vi "Get Highest Sub-Index.vi"(8 "Error In":errorcluster, 11 "reference in":refnum<class "OD Entry.lvclass">) -> (0 "Error Out":errorcluster, 2 "Highes Sub-Index":u8, 3 "reference out":refnum<class "OD Entry.lvclass">)   [LabVIEW 2024, in "EDS.lvlib" / "OD Entry.lvclass"]
doc: "Return max indicated subindex, or null if not array or record"
uses:
  OD Entry.lvclass
  OD Entry.lvclass/OD Entry.ctl
  Object Type.ctl
  EDS.lvlib
  Object Type/Object Type Base.lvclass
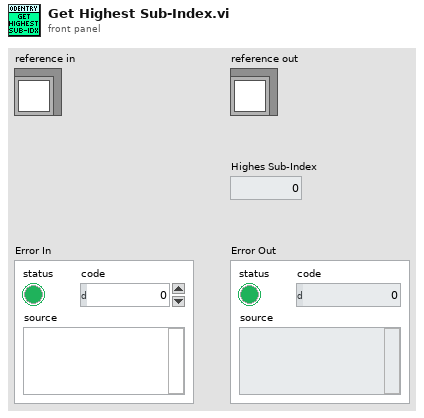
[diagram p1: front panel]
types:
  T1 = typedef "EDS.lvlib/Object Type.ctl" = u8
  T2 = typedef "EDS.lvlib/OD Entry.lvclass/ObjectAttributes.ctl" = cluster{"Index":u16, "ObjectType":refnum<class "Object Type Base.lvclass">, "Denotation":string, "Count":u8, "ObjExtend":u8, "PDOtype":T3, "Label":string, "Description":string, "Sub-Entries":map{u8, refnum<class "OD Sub-Entry.lvclass">}}
  T3 = typedef "EDS.lvlib/PDO Mapping Type.ctl" = enum16{"NO", "OPTIONAL", "RPDO", "TPDO", "DEFAULT"}
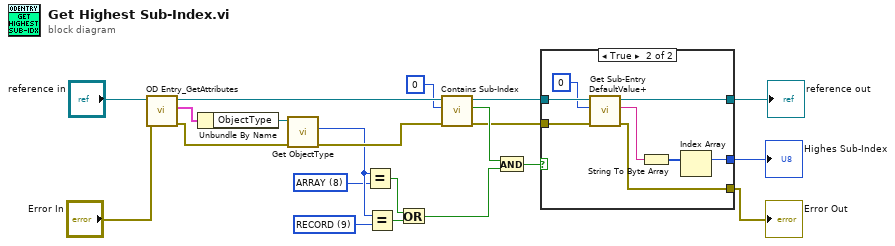
[diagram p0: block diagram]
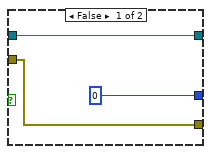
[diagram p2: hidden frame]
diagram:
  w1 = T1 9 items=["NULL"=0, "DOMAIN"=2, "DEFTYPE"=5, "DEFSTRUCT"=6, "VAR"=7, "ARRAY"=8, "RECORD"=9] ("ObjectType")
  w2 = T1 8 items=["NULL"=0, "DOMAIN"=2, "DEFTYPE"=5, "DEFSTRUCT"=6, "VAR"=7, "ARRAY"=8, "RECORD"=9] ("ObjectType")
  n1 = call "OD Entry_GetAttributes.vi"("Error In"="Error In", "reference in"="reference in") -> ("Error Out"=w5:errorcluster, "Data"=w18:T2, "reference out"=w19:refnum<class "OD Entry.lvclass">)  [unwired: 6 in, 1 out]
  n2 = Unbundle By Name(w18) -> ("ObjectType"=w16:refnum<class "Object Type Base.lvclass">)
  n3 = call-dynamic "Get ObjectType.vi"("error in"=w5, "Object Type in"=w16) -> ("error out"=w4:errorcluster, "ObjectType"=w3:T1)  [unwired: 6 in, 2 out]
  n4 = Equal?(x=w3, y=w2) -> (x = y?=w17:bool)
  n5 = Equal?(x=w3, y=w1) -> (x = y?=w13:bool)
  n6 = Or(x=w17, y=w13) -> (x .or. y?=w11:bool)
  n7 = call "Contains Sub-Index.vi"("Error In"=w4, "Sub-Index"=u16 0, "reference in"=w19) -> ("Error Out"=w7:errorcluster, "Contains?"=w12:bool, "reference out"=w15:refnum<class "OD Entry.lvclass">)  [unwired: 6 in]
  n8 = And(x=w12, y=w11) -> (x .and. y?=w9:bool)
  n9 = case shown="True" w9 {
    tunnel: w15 -> [w24 w32]
    tunnel: [w24 w31] -> w10
    tunnel: [u8 0 w27] -> w8
    tunnel: w7 -> [w22 w26]
    tunnel: [w22 w25] -> w6
    frame False {
    }
    frame True {
      n10 = call "Get Sub-Entry DefaultValue+.vi"("Error In"=w26, "Sub-Index"=u16 0, "reference in"=w32) -> ("Error Out"=w25:errorcluster, "DefaultValue"=w29:string, "reference out"=w31:refnum<class "OD Entry.lvclass">)  [unwired: 5 in, 1 out]
      n11 = String To Byte Array(string=w29) -> (unsigned byte array=w28:u8[])
      n12 = Index Array(array=w28) -> (element=w27:u8)  [unwired: 1 in]
    }
  }
  "Error Out" <- w6
  "reference out" <- w10
  "Highes Sub-Index" <- w8
